vi "FPGA Settings.vi"(6 "Action":T2, 8 "error in (no error)":errorcluster, 10 "FPGA Settings":T1={"Bitfile path"=path "", "RIO Device Address"="RIO0", "Group"=FALSE}, 11 "Item Ref":T3 format="%.0x") -> (0 "error out":errorcluster, 2 "FPGA Settings":T1, 3 "Item Ref out":T3=18446744073709551615 format="%.0x")   [LabVIEW 2019, in "FPGA Addon Shared.lvlib"]
uses:
  FPGA Addon Shared.lvlib
  Types/FPGA Settings.ctl
  <vilib>/NI VeriStand/Custom Device API/Custom Device Item Ref.ctl
  Types/FG Action.ctl
  Constants.vi
  <vilib>/NI VeriStand/Custom Device API/Get Item Property (Path).vi
  <vilib>/NI VeriStand/Custom Device API/Get Item Property (String).vi
  <vilib>/NI VeriStand/Custom Device API/Set Item Property (Path).vi
  <vilib>/NI VeriStand/Custom Device API/Set Item Property (String).vi
  <vilib>/NI VeriStand/Custom Device API/Custom Device API.lvlib
  <vilib>/NI VeriStand/Custom Device API/Get Item Property (Boolean).vi
  <vilib>/NI VeriStand/Custom Device API/Set Item Property (Boolean).vi
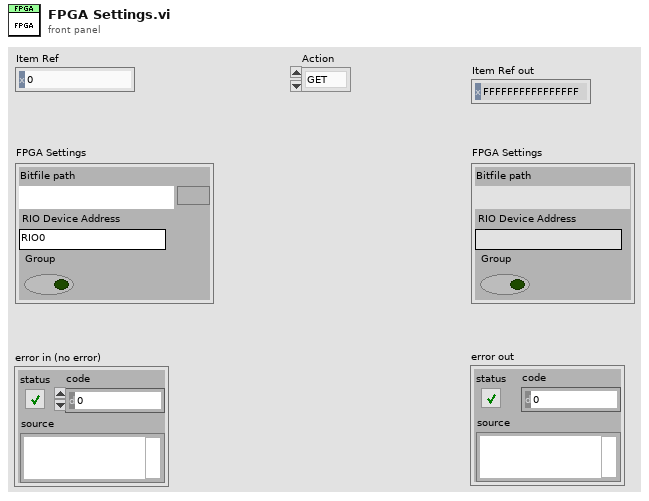
[diagram p1: front panel]
types:
  T1 = typedef "FPGA Addon Shared.lvlib/FPGA Settings.ctl" = cluster{"Bitfile path":path, "RIO Device Address":string, "Group":bool}
  T2 = typedef "FPGA Addon Shared.lvlib/FG Action.ctl" = enum8{"GET", "SET"}
  T3 = typedef "Custom Device API.lvlib/Custom Device Item Ref.ctl" = u64
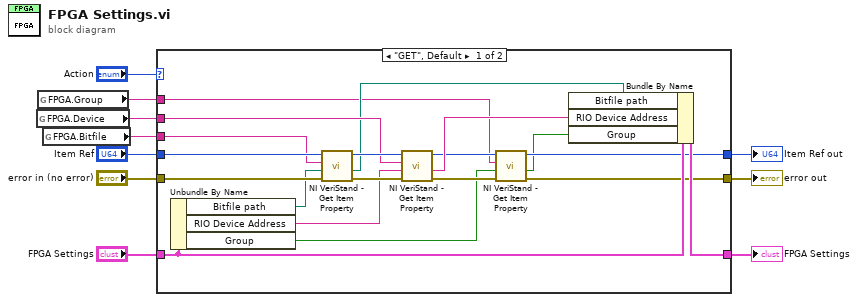
[diagram p0: block diagram]
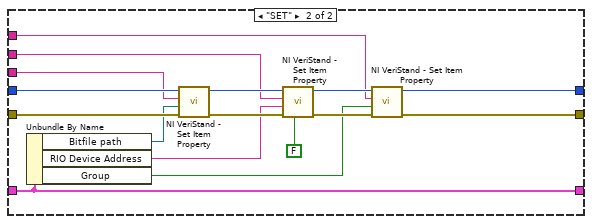
[diagram p2: hidden frame]
diagram:
  n1 = global read "Constants.vi" "FPGA.Device"() -> (w2:string)
  n2 = global read "Constants.vi" "FPGA.Group"() -> (w1:string)
  n3 = global read "Constants.vi" "FPGA.Bitfile"() -> (w4:string)
  n4 = case shown="\"GET\", Default" "Action" {
    tunnel: "error in (no error)" -> [w29 w45]
    tunnel: "Item Ref" -> [w28 w44]
    tunnel: "FPGA Settings" -> [w21 w42]
    tunnel: [w14 w34] -> w10
    tunnel: [w16 w32] -> w6
    tunnel: [w20 w42] -> w3
    tunnel: w4 -> [w27 w43]
    tunnel: w2 -> [w22 w36]
    tunnel: w1 -> [w11 w30]
    frame "GET", Default {
      n5 = Unbundle By Name(w21) -> ("Bitfile path"=w24:path, "RIO Device Address"=w23:string, "Group"=w13:bool)
      n6 = call-poly <vilib>:"NI VeriStand - Get Item Property.vi"("error in (no error)"=w29, "Default Value"=w24, "Property Name"=w27, "Item Ref in"=w28) -> ("error out"=w25:errorcluster, "Value"=w19:path, "Item Ref out"=w26:T3)  [unwired: 4 in, 1 out]
      n7 = call-poly <vilib>:"NI VeriStand - Get Item Property.vi"("error in (no error)"=w25, "Default Value"=w23, "Property Name"=w22, "Item Ref in"=w26) -> ("error out"=w15:errorcluster, "Value"=w18:string, "Item Ref out"=w17:T3)  [unwired: 4 in, 1 out]
      n8 = call-poly <vilib>:"NI VeriStand - Get Item Property.vi"("error in (no error)"=w15, "Default Value"=w13, "Property Name"=w11, "Item Ref in"=w17) -> ("error out"=w14:errorcluster, "Value"=w12:bool, "Item Ref out"=w16:T3)  [unwired: 4 in, 1 out]
      n9 = Bundle By Name(cluster=w21, "Bitfile path"=w19, "RIO Device Address"=w18, "Group"=w12) -> (w20:T1)
    }
    frame "SET" {
      n10 = Unbundle By Name(w42) -> ("Bitfile path"=w41:path, "RIO Device Address"=w37:string, "Group"=w31:bool)
      n11 = call-poly <vilib>:"NI VeriStand - Set Item Property.vi"("error in (no error)"=w45, "Value"=w41, "Property Name"=w43, "Item Ref in"=w44) -> ("error out"=w40:errorcluster, "Item Ref out"=w39:T3)  [unwired: 5 in, 1 out]
      n12 = call-poly <vilib>:"NI VeriStand - Set Item Property.vi"("Binary String (T)"=FALSE, "error in (no error)"=w40, "Value"=w37, "Property Name"=w36, "Item Ref in"=w39) -> ("error out"=w35:errorcluster, "Item Ref out"=w33:T3)  [unwired: 4 in, 1 out]
      n13 = call-poly <vilib>:"NI VeriStand - Set Item Property.vi"("error in (no error)"=w35, "Value"=w31, "Property Name"=w30, "Item Ref in"=w33) -> ("error out"=w34:errorcluster, "Item Ref out"=w32:T3)  [unwired: 5 in, 1 out]
    }
  }
  "error out" <- w10
  "Item Ref out" <- w6
  "FPGA Settings" <- w3
